vi "test_Series Configure.vi"(0 "error in (no error)":errorcluster) -> (8 "error out":errorcluster)   [LabVIEW 2023]
uses:
  Series/Series Base/Series Base.lvclass
panel:
  in  "HAL GOOP4:Series Base in":refnum<class "Series Base.lvclass">
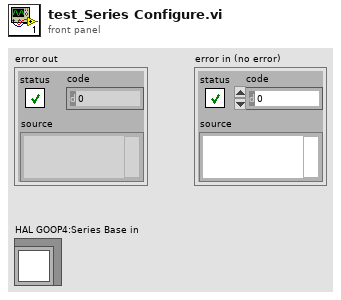
[diagram p1: front panel]
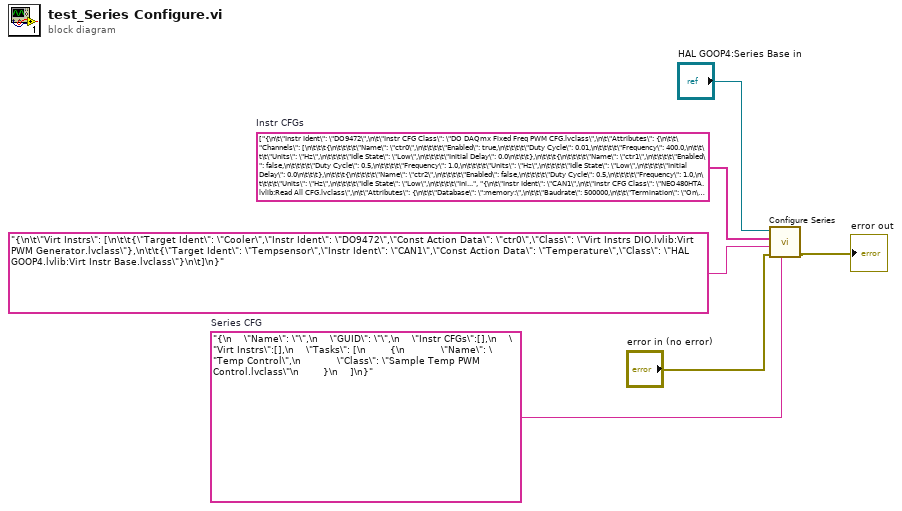
[diagram p0: block diagram]
diagram:
  w3 = "{\n    \"Name\": \"\",\n    \"GUID\": \"\",\n    \"Instr CFGs\":[],\n    \"Virt Instrs\":[],\n    \"Tasks\": [\n        {\n            \"Name\": \"Temp Control\",\n            \"Class\": \"Sample Temp PWM Control.lvclass\"\n        }\n    ]\n}"  # Series CFG
  w5 = string[] ["{\n\t\"Instr Ident\": \"DO9472\",\n\t\"Instr CFG Class\": \"DO DAQmx Fixed Freq PWM CFG.lvclass\",\n\t\"Attributes\": {\n\t\t\"Channels\": [\n\t\t\t{\n\t\t\t\t\"Name\": \"ctr0\",\n\t\t\t\t\"Enabled\": true,\n\t\t\t\t\"Duty Cycle\": 0.01,\n\t\t\t\t\"Frequency\": 400.0,\n\t\t\t\t\"Units\": \"Hz\",\n\t\t\t\t\"Idle State\": \"Low\",\n\t\t\t\t\"Initial Delay\": 0.0\n\t\t\t},\n\t\t\t{\n\t\t\t\t\"Name\": \"ctr1\",\n\t\t\t\t\"Enabled\": false,\n\t\t\t\t\"Duty Cycle\": 0.5,\n\t\t\t\t\"Frequency\": 1.0,\n\t\t\t\t\"Units\": \"Hz\",\n\t\t\t\t\"Idle State\": \"Low\",\n\t\t\t\t\"Initial Delay\": 0.0\n\t\t\t},\n\t\t\t{\n\t\t\t\t\"Name\": \"ctr2\",\n\t\t\t\t\"Enabled\": false,\n\t\t\t\t\"Duty Cycle\": 0.5,\n\t\t\t\t\"Frequency\": 1.0,\n\t\t\t\t\"Units\": \"Hz\",\n\t\t\t\t\"Idle State\": \"Low\",\n\t\t\t\t\"Initial Delay\": 0.0\n\t\t\t},\n\t\t\t{\n\t\t\t\t\"Name\": \"ctr3\",\n\t\t\t\t\"Enabled\": false,\n\t\t\t\t\"Duty Cycle\": 0.5,\n\t\t\t\t\"Frequency\": 1.0,\n\t\t\t\t\"Units\": \"Hz\",\n\t\t\t\t\"Idle State\": \"Low\",\n\t\t\t\t\"Initial Delay\": 0.0\n\t\t\t}\n\t\t],\n\t\t\"Timing\": {\n\t\t\t\"Samples per Channel\": 1000,\n\t\t\t\"Sample Mode\": \"Continuous Samples\",\n\t\t\t\"Sample Rate\": 0.0,\n\t\t\t\"Sample Clock Source\": \"Implicit\",\n\t\t\t\"Active Edge\": \"Rising\"\n\t\t},\n\t\t\"Trigger\": {\n\t\t\t\"Trigger Type\": \"No Trigger\"\n\t\t}\n\t}\n}", "{\n\t\"Instr Ident\": \"CAN1\",\n\t\"Instr CFG Class\": \"NEO480HTA.lvlib:Read All CFG.lvclass\",\n\t\"Attributes\": {\n\t\t\"Database\": \":memory:\",\n\t\t\"Baudrate\": 500000,\n\t\t\"Termination\": \"On\",\n\t\t\"CAN Frames\": [\n\t\t\t{\n\t\t\t\t\"Frame name\": \"Dew Point\",\n\t\t\t\t\"Identifier\": 1152,\n\t\t\t\t\"Extended Identifier\": false,\n\t\t\t\t\"Payload Length\":8,\n\t\t\t\t\"Timing Type\":\"Event Data\",\n\t\t\t\t\"Transmit Time\":0,\n\t\t\t\t\"Comment\":\"\"\n\t\t\t},\n\t\t\t{\n\t\t\t\t\"Frame name\": \"Dew Point Raw\",\n\t\t\t\t\"Identifier\": 1153,\n\t\t\t\t\"Extended Identifier\": false,\n\t\t\t\t\"Payload Length\":8,\n\t\t\t\t\"Timing Type\":\"Event Data\",\n\t\t\t\t\"Transmit Time\":0,\n\t\t\t\t\"Comment\":\"\"\n\t\t\t}\n\t\t],\n\t\t\"Acquire\": {\n\t\t\t\"Type\": \"Read Frame\"\n\t\t}\n\t}\n}"]  # Instr CFGs
  n1 = call "Configure Series.vi"("Series CFG"=w3, "error in (no error)"="error in (no error)", "Virt Instrs CFG"="{\n\t\"Virt Instrs\": [\n\t\t{\"Target Ident\": \"Cooler\",\"Instr Ident\": \"DO9472\",\"Const Action Data\": \"ctr0\",\"Class\": \"Virt Instrs DIO.lvlib:Virt PWM Generator.lvclass\"},\n\t\t{\"Target Ident\": \"Tempsensor\",\"Instr Ident\": \"CAN1\",\"Const Action Data\": \"Temperature\",\"Class\": \"HAL GOOP4.lvlib:Virt Instr Base.lvclass\"}\n\t]\n}", "Instr CFGs"=w5, "HAL GOOP4:Series Base in"="HAL GOOP4:Series Base in") -> ("error out"=→"error out":errorcluster)  [unwired: 5 in, 1 out]
